vi "test_00_temp.vi"() -> ()   [LabVIEW 2015]
uses:
  <userlib>/antonio-alexander/lv-waitgroup/lv-waitgroup.lvlib
panel:
  in  "skip_done":bool
  in  "do_it_button":bool
  in  "stop":bool
  in  "timeout_ms":i32=100
  in  "wait_time_ms":u32=5000
  in  "add_timeout_ms":i32
  out "active_processes":i32
  out "processes_remaining []":i32[](array[numeric])
  in  "max_processes":i32=5
  out "error out":errorcluster
  # "This example is meant to show how lv-waitgroup can be\nused to limit and/or keep track of asynchronously running\nprocesses/threads.  This is VERY similar if not identical to\nworker pools.\n\n1. Set the maximum number of simultaneous processes\n2. Start the VI\n3. Use the add_timeous_ms control to set how long to\n    attempt to add a processes\n3. Use the \"DO IT\" button to start an asynchronous process\n4. Enable \"Skip Done\" to tell the wait.vi not to return cleanly\n5. Click the STOP button to stop the example"
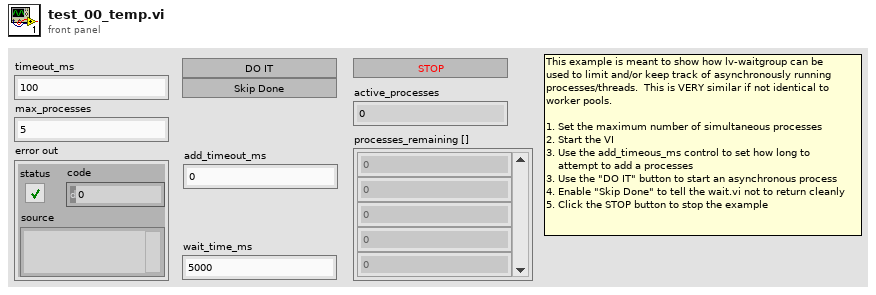
[diagram p1: front panel]
types:
  T1 = typedef "lv-waitgroup.lvlib/api_waitgroup.ctl" = cluster{"waitgroups":refnum<data-value>, "waitgroup":string}
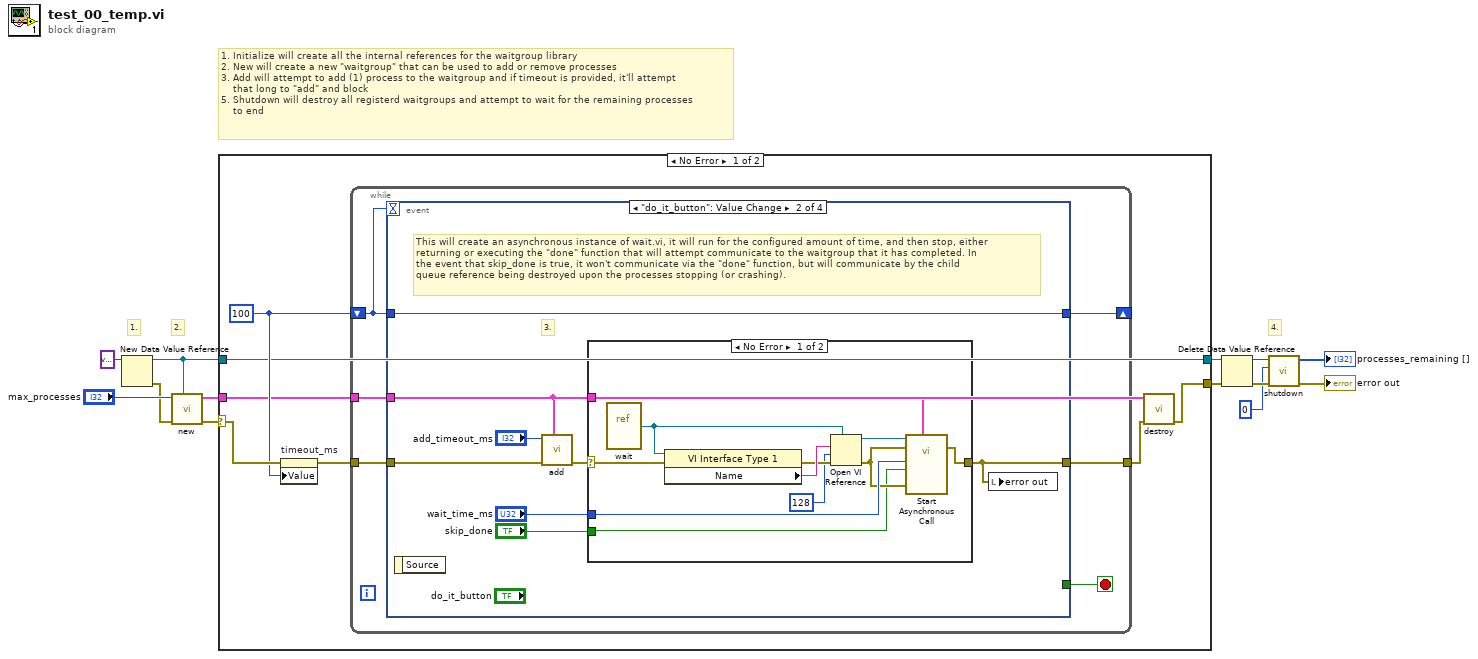
[diagram p0: block diagram]
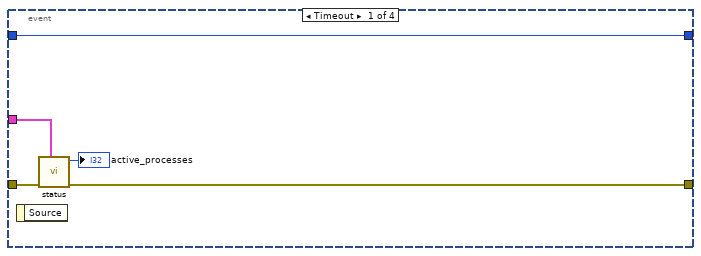
[diagram p2: hidden frame]
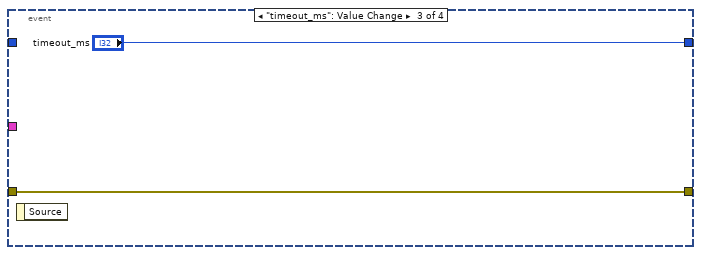
[diagram p4: hidden frame]
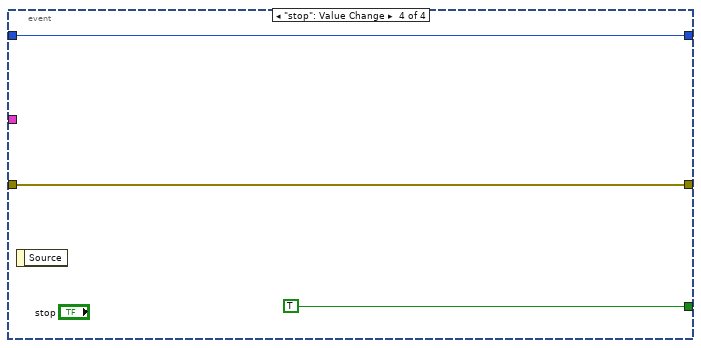
[diagram p5: hidden frame]
diagram:
  # "1. Initialize will create all the internal references for the waitgroup library\n2. New will create a new \"waitgroup\" that can be used to add or remove processes\n3. Add will attempt to add (1) process to the waitgroup and if timeout is provided, it'll attempt\n    that long to \"add\" and block\n5. Shutdown will destroy all registerd waitgroups and attempt to wait for the remaining processes\n    to end"
  # "4."
  # "2."
  # "1."
  n1 = New Data Value Reference(data value=variant) -> (data value reference=w8:refnum<data-value>, error out=w5:errorcluster)  [unwired: 1 in]
  n2 = call <userlib>:"new.vi"("waitgroups"=w8, "error in (no error)"=w5, "max_waitgroup_processes"="max_processes") -> ("error out"=w1:errorcluster, "waitgroup"=w2:T1)  [unwired: 7 in]
  n3 = case shown="No Error" w1 {
    selector: w1 -> [w20 w57]
    tunnel: w2 -> [w16 _]
    tunnel: w8 -> [w17 w58]
    tunnel: [w17 w58] -> w11
    tunnel: [w14 w57] -> w12
    frame No Error {
      w19 = 100 ("timeout_ms 2")
      n4 = property on="timeout_ms" class="DigNum (strict)"(error in=w20, "Value"=w19) -> (error out=w18:errorcluster)  [unwired: 1 in, 1 out]
      n5 = while {
        tunnel: w18 -> [w25]
        tunnel: [w23] -> w15
        tunnel: w16 -> [w24]
        shift-right: [w21] -> _
        shift-left: w19 -> [w22]
        stop <- w26 stop-if-true
        n6 = event shown="[1] \"do_it_button\": Value Change" {
          selector: _ -> [_ _ _ _]
          dyn-events: _ -> [_ _ _ _]
          timeout: w22 -> [_ _ _ _]
          tunnel: [_ _ _ TRUE] -> w26
          tunnel: w25 -> [w30 w38 w52 w55]
          tunnel: [w29 w32 w52 w55] -> w23
          tunnel: w24 -> [w28 w36 _ _]
          tunnel: w22 -> [w27 w33 _ w54]
          tunnel: [w27 w33 "timeout_ms" w54] -> w21
          event Timeout {
            n7 = event-data() -> ()  [unwired: 1 in, 1 out]
            n8 = call <userlib>:"status.vi"("waitgroup"=w28, "error in (no error)"=w30) -> ("error out"=w29:errorcluster, "active"=→"active_processes":i32)  [unwired: 8 in]
          }
          event "do_it_button": Value Change {
            # "This will create an asynchronous instance of wait.vi, it will run for the configured amount of time, and then stop, either\nreturning or executing the \"done\" function that will attempt communicate to the waitgroup that it has completed. In\nthe event that skip_done is true, it won't communicate via the \"done\" function, but will communicate by the child\nqueue reference being destroyed upon the processes stopping (or crashing)."
            # "3."
            n9 = event-data() -> ()  [unwired: 1 in, 1 out]
            n10 = call <userlib>:"add.vi"("waitgroup"=w36, "error in (no error)"=w38, "timeout_ms"="add_timeout_ms") -> ("error out"=w37:errorcluster)  [unwired: 8 in]
            n11 = case shown="No Error" w37 {
              selector: w37 -> [w43 w51]
              tunnel: "wait_time_ms" -> [w45 _]
              tunnel: [w44 w51] -> w32
              tunnel: w36 -> [w42 _]
              tunnel: "skip_done" -> [w40 _]
              frame No Error {
                n12 = vi-ref <userlib>:"wait.vi"() -> (w49:refnum<vi>)
                n13 = property class="VI Interface Type 1"(reference=w49, error in=w43) -> (error out=w48:errorcluster, "Name"=w50:string)  [unwired: 1 out]
                n14 = Open VI Reference(type specifier VI Refnum (for type only)=w49, vi path=w50, options=128, error in (no error)=w48) -> (vi reference=w47:refnum<vi>, error out=w41:errorcluster)  [unwired: 2 in]
                n15 = call-by-ref "Start Asynchronous Call"(reference=w47, error in=w41, "waitgroup"=w42, 8:"error in (no error)"=w41, "skip_done"=w40, "wait_ms"=w45) -> (error out=w44:errorcluster)  [unwired: 7 in, 2 out]
              }
              frame Error {
              }
            }
            n16 = local write "error out"(w32) -> ()
          }
          event "timeout_ms": Value Change {
            n17 = event-data() -> ()  [unwired: 1 in, 1 out]
          }
          event "stop": Value Change {
            n18 = event-data() -> ()  [unwired: 1 in, 1 out]
          }
        }
      }
      n19 = call <userlib>:"destroy.vi"("error in (no error)"=w15, "waitgroup"=w16) -> ("error out"=w14:errorcluster)  [unwired: 8 in, 1 out]
    }
    frame Error {
    }
  }
  n20 = Delete Data Value Reference(data value reference=w11, error in=w12) -> (data value=w9:variant, error out=w10:errorcluster)
  n21 = call <userlib>:"shutdown.vi"("error in (no error)"=w10, "wait_ms"=0, "waitgroups"=w9) -> ("error out"=→"error out":errorcluster, "processes_remaining []"=→"processes_remaining []":i32[])  [unwired: 7 in]
